vi "Query Calibration kits.vi"(8 "error in (no error)":errorcluster, 10 "Connector type":T1(ring), 11 "VNA-CMT S2 S4 in":refnum<class "VNA-CMT S2 S4.lvclass">) -> (0 "error out":errorcluster, 2 "Cal kits installed":string[](array[string]), 3 "VNA-CMT S2 S4 out":refnum<class "VNA-CMT S2 S4.lvclass">)   [LabVIEW 2020, in "VNA-CMT S2 S4.lvclass"]
doc: "Queryes the calibration kits installed on the VNA dependent on connector type.\nIf the VNA support E-cal it reports this aswell as the first sting in the array."
uses:
  VNA-CMT S2 S4.lvclass
  C:/Sandbox/Git_Sandbox/WiSpry Test Framework source code (LV20)/WiSpry Test Framework/Instruments/Instrument.lvclass
  Instrument.lvclass/Instrument.ctl
  Instrument.lvclass
  <instrlib>/CMT S2 and S4 VNA/CMT S2 and S4 VNA.lvlib
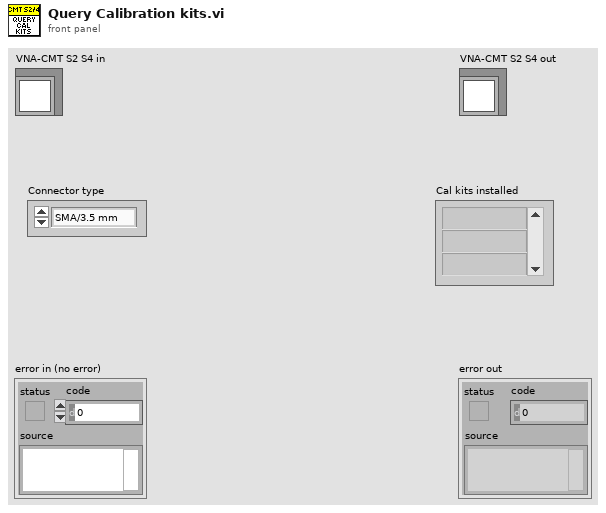
[diagram p1: front panel]
types:
  T1 = enum16{"SMA/3.5 mm", "2.92 mm", "2.4 mm", "1.85 mm", "N 50 Ohm", "N 75 Ohm", "7-16"}
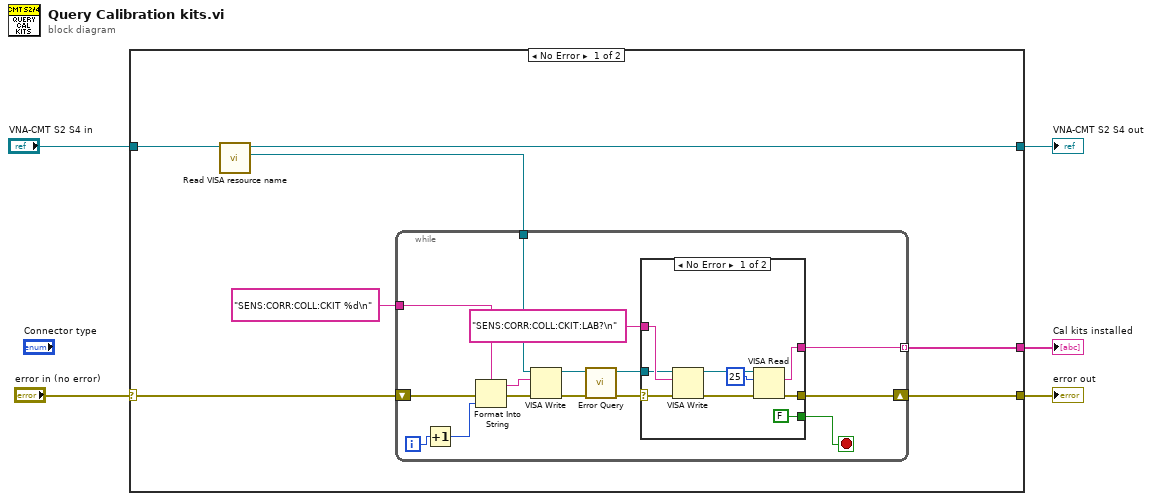
[diagram p0: block diagram]
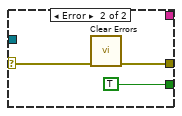
[diagram p2: hidden frame]
diagram:
  n1 = case shown="No Error" "error in (no error)" {
    selector: "error in (no error)" -> [w10 w40]
    tunnel: "VNA-CMT S2 S4 in" -> [w12 w41]
    tunnel: [w11 w41] -> w4
    tunnel: [w9 w40] -> w5
    tunnel: [w6 _] -> w1
    frame No Error {
      n2 = call "Read VISA resource name.vi"("Instrument in"=w12) -> ("VISA resource name"=w8:refnum<visa-resource-name>, "Instrument out"=w11:refnum<class "VNA-CMT S2 S4.lvclass">)  [unwired: 9 in]
      n3 = while {
        shift-right: [w26] -> w9
        shift-left: w10 -> [w25]
        tunnel: w8 -> [w23]
        tunnel: "SENS:CORR:COLL:CKIT %d\n" ("write buffer") -> [w21]
        tunnel: [w14] -> w6 mode=indexing
        i -> [w20]
        stop <- w15 stop-if-true
        n4 = Increment(x=w20) -> (x+1=w19:i32)
        n5 = Format Into String(format string=w21, error in=w25, w19) -> (resulting string=w24:string, error out=w22:errorcluster)  [unwired: 1 in]
        n6 = VISA Write(VISA resource name=w23, write buffer=w24, error in (no error)=w22) -> (VISA resource name out=w17:refnum<visa-resource-name>, error out=w18:errorcluster)  [unwired: 1 out]
        n7 = call <instrlib>:"Error Query.vi"("error in (no error)"=w18, "VISA resource name"=w17) -> ("error out"=w16:errorcluster, "VISA resource name out"=w13:refnum<visa-resource-name>)  [unwired: 6 in, 2 out]
        n8 = case shown="No Error" w16 {
          selector: w16 -> [w30 w39]
          tunnel: "SENS:CORR:COLL:CKIT:LAB?\n" ("write buffer") -> [w36 _]
          tunnel: [w32 w38] -> w26
          tunnel: [FALSE TRUE] -> w15
          tunnel: [w29 _] -> w14
          tunnel: w13 -> [w28 _]
          frame No Error {
            n9 = VISA Write(VISA resource name=w28, write buffer=w36, error in (no error)=w30) -> (VISA resource name out=w35:refnum<visa-resource-name>, error out=w33:errorcluster)  [unwired: 1 out]
            n10 = VISA Read(VISA resource name=w35, byte count=u32 25, error in (no error)=w33) -> (read buffer=w29:string, error out=w32:errorcluster)  [unwired: 2 out]
          }
          frame Error {
            n11 = call <vilib>:"Clear Errors.vi"("error in (no error)"=w39) -> ("error out"=w38:errorcluster)  [unwired: 5 in, 1 out]
          }
        }
      }
    }
    frame Error {
    }
  }
  "error out" <- w5
  "VNA-CMT S2 S4 out" <- w4
  "Cal kits installed" <- w1
